vi "Get Behavior Flags.vi"(8 "error in (no error)":errorcluster, 11 "Element in":refnum<class "Element.lvclass">) -> (0 "error out":errorcluster, 2 "Behavior":T1={"Children"=enum."Multiple", "Editable"=TRUE, "XML uses />"=FALSE}, 3 "Element out":refnum<class "Element.lvclass">)   [LabVIEW 2026, in "VILab.lvlib" / "Element.lvclass"]
uses:
  Element.lvclass
  Element.lvclass/Element.ctl
  Data Item/Child Support.ctl
  Data Item/Data Item.lvclass
  Data Item/Behavior Flags.ctl
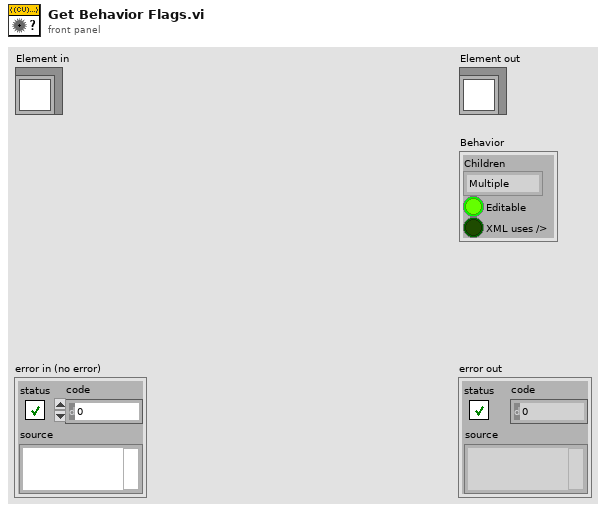
[diagram p1: front panel]
types:
  T1 = typedef "VILab.lvlib/Data Item.lvclass/Behavior Flags.ctl" = cluster{"Children":T2, "Editable":bool, "XML uses />":bool}
  T2 = typedef "VILab.lvlib/Data Item.lvclass/Child Support.ctl" = enum16{"None", "One", "At most one", "Multiple"}
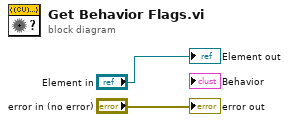
[diagram p0: block diagram]
diagram:
  "error out" <- "error in (no error)"
  "Element out" <- "Element in"
